vi "Write Nodes.vi"(8 "error in (no error)":errorcluster, 10 "Nodes":refnum<class "Messenger.lvclass">[](array[class]), 11 "Messenger Composite in":refnum<class "Messenger Composite.lvclass">) -> (0 "error out":errorcluster, 3 "Messenger Composite out":refnum<class "Messenger Composite.lvclass">)   [LabVIEW 2024, in "Messenger Composite.lvclass"]
uses:
  Messenger Composite.lvclass
  Messenger/Messenger.lvclass
  Messenger Composite.lvclass/Messenger Composite.ctl
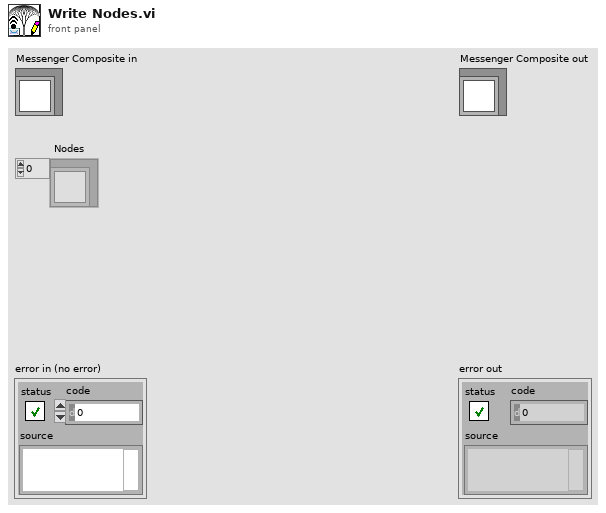
[diagram p1: front panel]
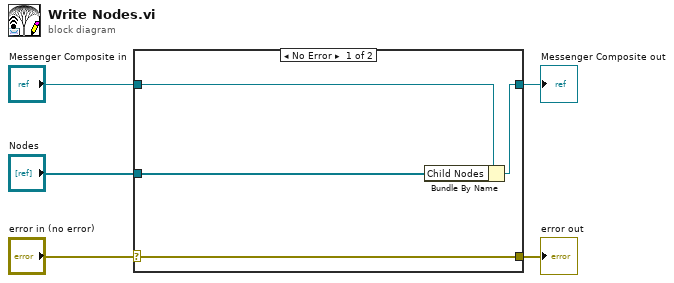
[diagram p0: block diagram]
diagram:
  n1 = case shown="No Error" "error in (no error)" {
    selector: "error in (no error)" -> [w9 w10]
    tunnel: [w9 w10] -> w4
    tunnel: [w7 w11] -> w2
    tunnel: "Messenger Composite in" -> [w8 w11]
    tunnel: "Nodes" -> [w6 _]
    frame No Error {
      n2 = Bundle By Name(cluster=w8, "Child Nodes"=w6) -> (w7:refnum<class "Messenger Composite.lvclass">)
    }
    frame Error {
    }
  }
  "error out" <- w4
  "Messenger Composite out" <- w2
